vi "CALIBRATE 2016.vi"(0 "flow_slope_IN":dbl=51.35 format="%.2f", 1 "Array in":refnum<k24>[](array[refnum]), 5 "pressure_slope_IN":dbl=23.33 format="%.2f", 7 "Descriptions":string[](array[string]), 9 "string_pot_slope_IN":dbl=1.5 format="%.2f", 11 "error in (no error)":errorcluster, 12 "Sensor Cluster":T1, 14 "Path":path=path "C:/KPRO_2010/Output_files/slopes-cal-record.txt") -> (2 "Array out":refnum<k24>[](array[refnum]), 4 "flow_slope_OUT":dbl=51.35 format="%.2f", 6 "pressure_slope_OUT":dbl=23.33 format="%.2f", 10 "string_pot_slope_OUT":dbl=1.5 format="%.2f", 13 "Sensor Cluster 2":T1, 15 "error out":errorcluster)   [LabVIEW 2016]
uses:
  Waterloo DAQ/controls/MCC DAQ Readings.ctl
  C:/Program Files (x86)/National Instruments/LabVIEW 2016/vi.lib/ULx/ULx_LV.dll
panel:
  in  "exit":bool
  in  "string_pot":bool
  in  "pressure":bool
  in  "flow":bool
  in  "start path":path=path "C:/"
  in  "all":bool
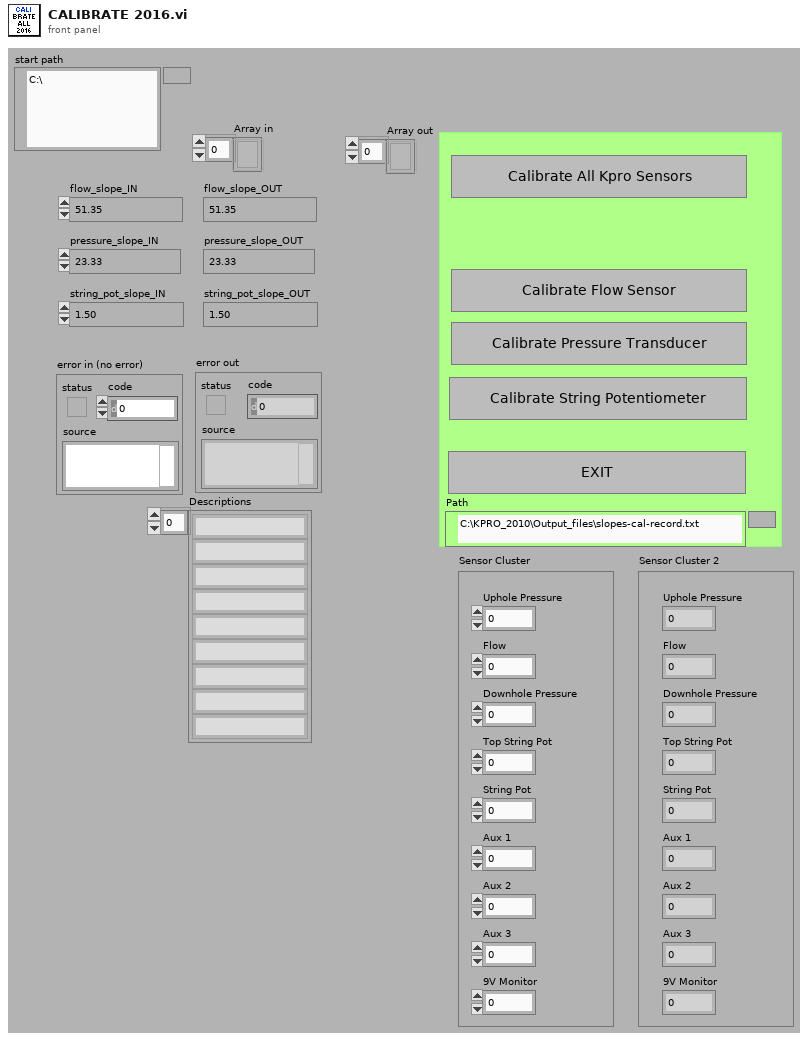
[diagram p1: front panel]
types:
  T1 = typedef "MCC DAQ Readings.ctl" = cluster{"Uphole Pressure":dbl, "Flow":dbl, "Downhole Pressure":dbl, "Top String Pot":dbl, "String Pot":dbl, "Aux 1":dbl, "Aux 2":dbl, "Aux 3":dbl, "9V Monitor":dbl}
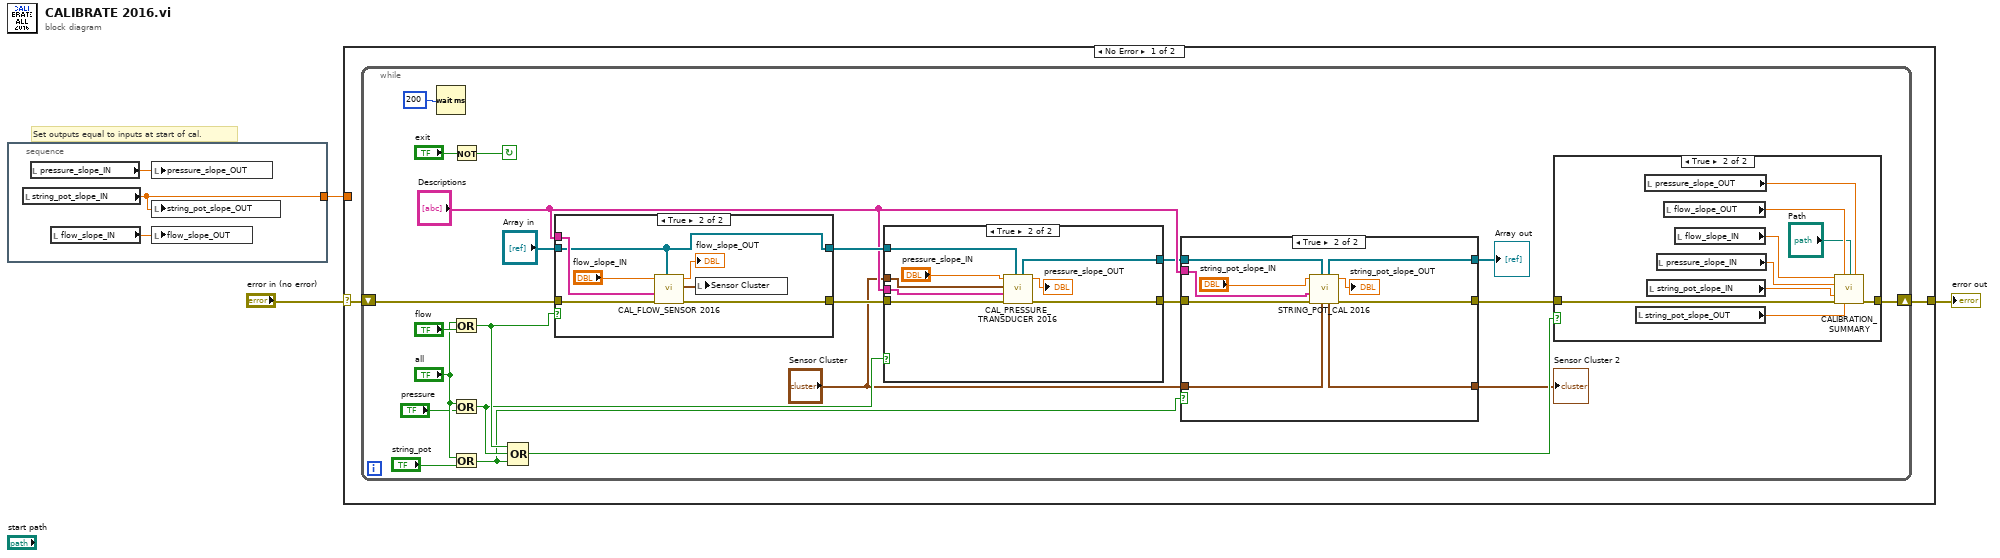
[diagram p0: block diagram]
diagram:
  # "Set outputs equal to inputs at start of cal."
  n1 = stacked-sequence {
    tunnel: [w4] -> w1
    frame #0 {
      n2 = local read "string_pot_slope_IN"() -> (w4:dbl)
      n3 = local read "pressure_slope_IN"() -> (w5:dbl)
      n4 = local read "flow_slope_IN"() -> (w6:dbl)
      n5 = local write "pressure_slope_OUT"(w5) -> ()
      n6 = local write "string_pot_slope_OUT"(w4) -> ()
      n7 = local write "flow_slope_OUT"(w6) -> ()
    }
  }
  n8 = case shown="No Error" "error in (no error)" {
    selector: "error in (no error)" -> [w8 w73]
    tunnel: [w7 w73] -> w2
    tunnel: w1 -> [_ _]
    frame No Error {
      n9 = while {
        shift-left: w8 -> [w28]
        shift-right: [w20] -> w7
        stop <- w31 continue-if-true
        n10 = Wait (ms)(milliseconds to wait=u32 200) -> ()  [unwired: 1 out]
        n11 = Not(x="exit") -> (.not. x?=w31:bool)
        n12 = Or(x="all", y="flow") -> (x .or. y?=w19:bool)
        n13 = Or(x="all", y="pressure") -> (x .or. y?=w18:bool)
        n14 = Or(x="all", y="string_pot") -> (x .or. y?=w17:bool)
        n15 = Compound Arithmetic op=OR(w19, w18, w17) -> (w16:bool)
        n16 = case shown="True" w19 {
          tunnel: w28 -> [w65 w72]
          tunnel: [w65 w71] -> w25
          tunnel: "Descriptions" -> [_ w68]
          tunnel: "Array in" -> [w64 w67]
          tunnel: [w64 w67] -> w14
          frame False {
          }
          frame True {
            n17 = call "CAL_FLOW_SENSOR 2016.vi"("Array in"=w67, "error in (no error)"=w72, "Descriptions"=w68, "flow_slope_IN"="flow_slope_IN") -> ("error out"=w71:errorcluster, "Sensor Cluster"=w66:T1, "flow_slope_OUT"=→"flow_slope_OUT":dbl)  [unwired: 4 in, 1 out]
            n18 = local write "Sensor Cluster"(w66) -> ()
          }
        }
        n19 = case shown="True" w18 {
          tunnel: [w55 w62] -> w26
          tunnel: w25 -> [w55 w63]
          tunnel: "Sensor Cluster" -> [_ w59]
          tunnel: "Descriptions" -> [_ w58]
          tunnel: w14 -> [w54 w57]
          tunnel: [w54 w56] -> w11
          frame False {
          }
          frame True {
            n20 = call "CAL_PRESSURE_TRANSDUCER 2016.vi"("Array in"=w57, "error in (no error)"=w63, "Descriptions"=w58, "Sensor Cluster"=w59, "pressure_slope_IN"="pressure_slope_IN") -> ("error out"=w62:errorcluster, "pressure_slope_OUT"=→"pressure_slope_OUT":dbl, "Array out"=w56:refnum<k24>[])  [unwired: 3 in, 1 out]
          }
        }
        n21 = case shown="True" w17 {
          tunnel: w26 -> [w44 w47]
          tunnel: [w44 w46] -> w21
          tunnel: "Descriptions" -> [_ w53]
          tunnel: "Sensor Cluster" -> [w43 w52]
          tunnel: w11 -> [w42 w51]
          tunnel: [w42 w50] -> w10
          tunnel: [w43 w45] -> w9
          frame False {
          }
          frame True {
            n22 = call "STRING_POT_CAL 2016.vi"("Sensor Cluster"=w52, "Array in"=w51, "error in (no error)"=w47, "Descriptions"=w53, "string_pot_slope_IN"="string_pot_slope_IN") -> ("error out"=w46:errorcluster, "string_pot_slope_OUT"=→"string_pot_slope_OUT":dbl, "Sensor Cluster 2"=w45:T1, "Array out"=w50:refnum<k24>[])  [unwired: 3 in]
          }
        }
        "Array out" <- w10
        "Sensor Cluster 2" <- w9
        n23 = case shown="True" w16 {
          tunnel: w21 -> [w32 w41]
          tunnel: [w32 w40] -> w20
          frame False {
          }
          frame True {
            n24 = local read "string_pot_slope_OUT"() -> (w34:dbl)
            n25 = local read "pressure_slope_OUT"() -> (w39:dbl)
            n26 = local read "string_pot_slope_IN"() -> (w35:dbl)
            n27 = local read "pressure_slope_IN"() -> (w36:dbl)
            n28 = local read "flow_slope_OUT"() -> (w38:dbl)
            n29 = local read "flow_slope_IN"() -> (w37:dbl)
            n30 = call "CALIBRATION_SUMMARY.vi"("flow_slope_IN"=w37, "flow_slope_OUT"=w38, "Path"="Path", "pressure_slope_OUT"=w39, "pressure_slope_IN"=w36, "string_pot_slope_IN"=w35, "error in (no error)"=w41, "string_pot_slope_OUT"=w34) -> ("error out"=w40:errorcluster)  [unwired: 7 in]
          }
        }
      }
    }
    frame Error {
    }
  }
  "error out" <- w2
